vi "Wind Turbine Simulation - One Cluster.vi"() -> (0 "Cluster":T2)   [LabVIEW 2009]
doc: "This is a cluster for a Wind Turbine template.\n\nAAL 9/09"
uses:
  Controls/File Type.ctl
  Wind Report/Wind Report.lvclass
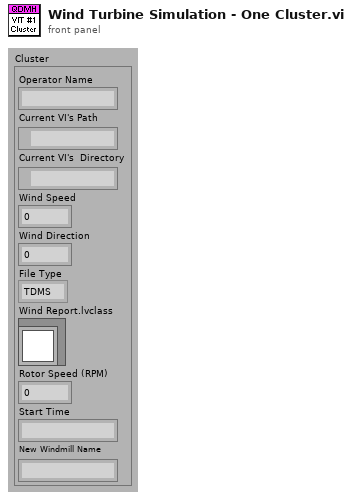
[diagram p1: front panel]
types:
  T1 = typedef "File Type.ctl" = enum16{"TDMS", "TXT"}
  T2 = cluster{"Operator Name":string, "Current VI's Path":path, "Current VI's  Directory":path, "Wind Speed":dbl, "Wind Direction":dbl, "File Type":T1, "Wind Report.lvclass":refnum<class "Wind Report.lvclass">, "Rotor Speed (RPM)":dbl, "Start Time":string, "New Windmill Name":string}
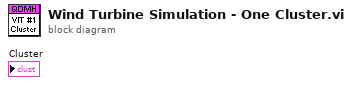
[diagram p0: block diagram]
diagram:
